vi "ReadSRIMSimulationFile.vi"(8 "Error In":errorcluster, 11 "SRIM Simulation File Path":path) -> (0 "Error Out":errorcluster, 3 "Collision Events":cluster{"Depth":dbl[], "DPA":dbl[]})   [LabVIEW 2012]
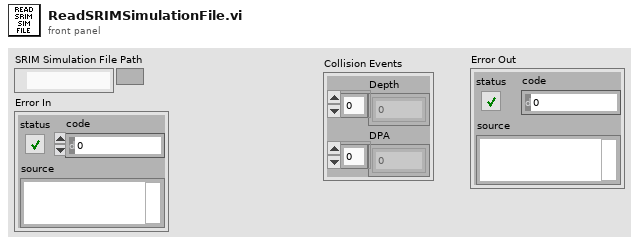
[diagram p1: front panel]
types:
  T1 = enum16{"open", "replace", "create", "open or create", "replace or create", "replace or create with confirmation"}
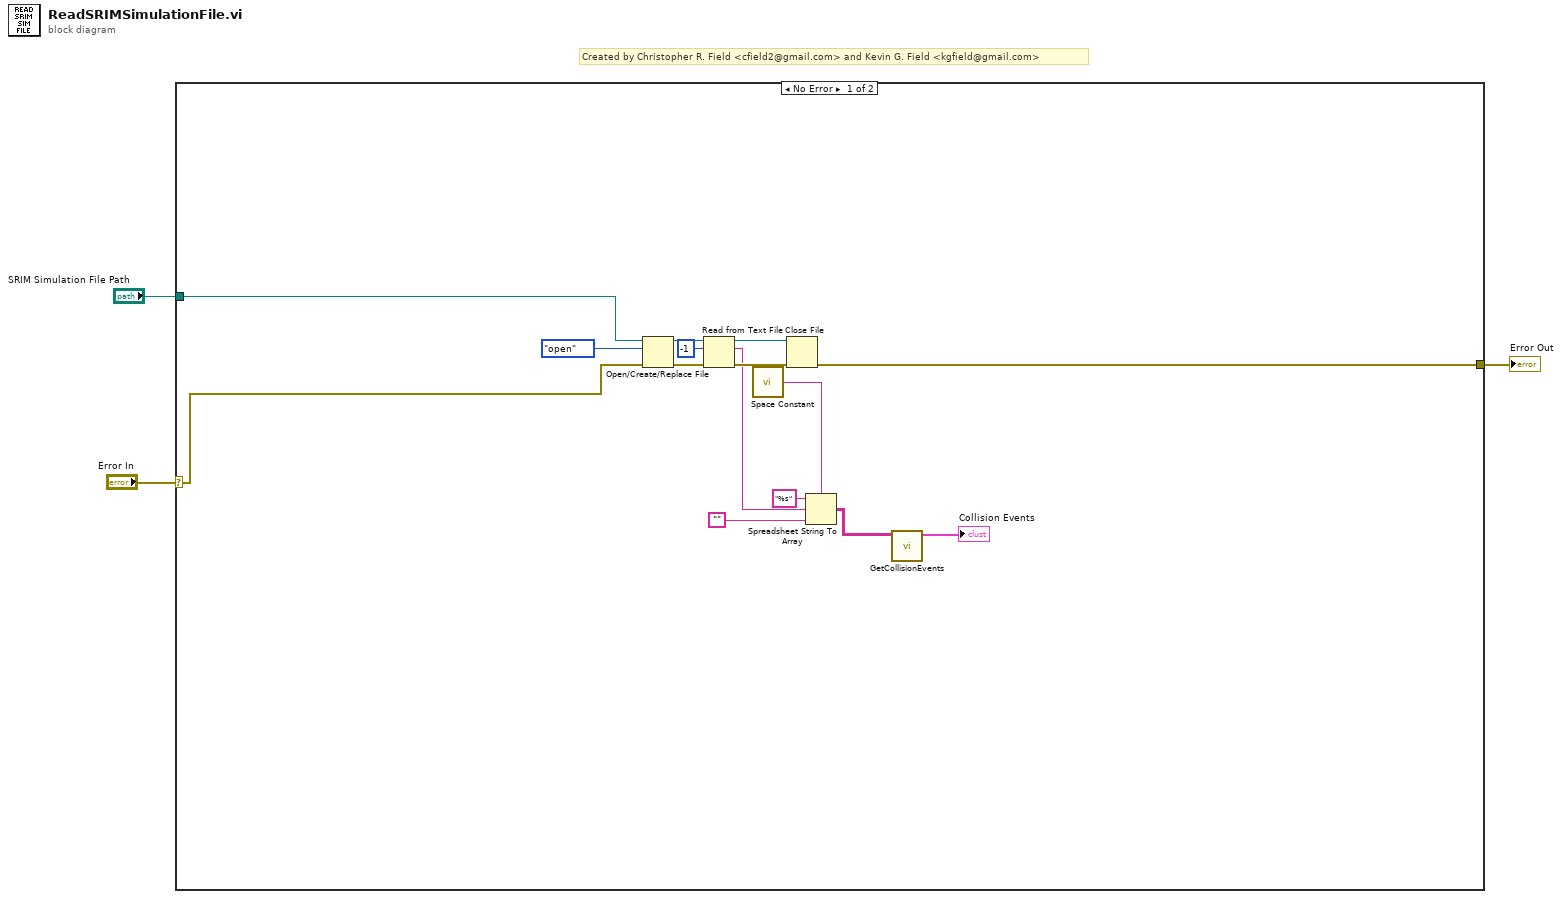
[diagram p0: block diagram]
diagram:
  # "Created by Christopher R. Field <cfield2@gmail.com> and Kevin G. Field <kgfield@gmail.com>"
  n1 = case shown="No Error" "Error In" {
    selector: "Error In" -> [w7 w19]
    tunnel: "SRIM Simulation File Path" -> [w8 _]
    tunnel: [w6 w19] -> w1
    frame No Error {
      n2 = Open/Create/Replace File(file path (use dialog)=w8, error in=w7, operation (0:open)=T1."open") -> (refnum out=w17:refnum<file>, error out=w16:errorcluster)  [unwired: 3 in, 1 out]
      n3 = Read from Text File(file (use dialog)=w17, count=-1, error in=w16) -> (refnum out=w15:refnum<file>, text=w12:string, error out=w14:errorcluster)  [unwired: 1 in, 1 out]
      n4 = call <vilib>:"Space Constant.vi"() -> ("String"=w9:string)
      n5 = Close File(refnum=w15, error in=w14) -> (error out=w6:errorcluster)  [unwired: 1 out]
      n6 = Spreadsheet String To Array(delimiter (Tab)=w9, format string="%s", spreadsheet string=w12, array type (2D Dbl)="") -> (array=w5:string[][])
      n7 = call "GetCollisionEvents.vi"("Tab Array"=w5) -> ("Collision Events"=→"Collision Events":cluster{"Depth":dbl[], "D1":dbl[]})  [unwired: 10 in]
    }
    frame Error {
    }
  }
  "Error Out" <- w1
